vi "testCmdLineParser.vi"(8 "error in (no error)":errorcluster) -> (0 "error out":errorcluster)   [LabVIEW 2018]
uses:
  <vilib>/addons/_JKI Toolkits/Caraya/classes/Assert/Assert False.vi
  <vilib>/addons/_JKI Toolkits/Caraya/classes/Assert/Assert True.vi
  <vilib>/addons/_JKI Toolkits/Caraya/classes/Test/Test.lvclass
  <vilib>/addons/_JKI Toolkits/Caraya/classes/Assert/Assert.lvclass
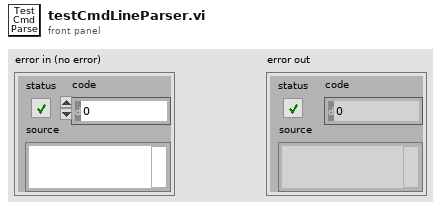
[diagram p1: front panel]
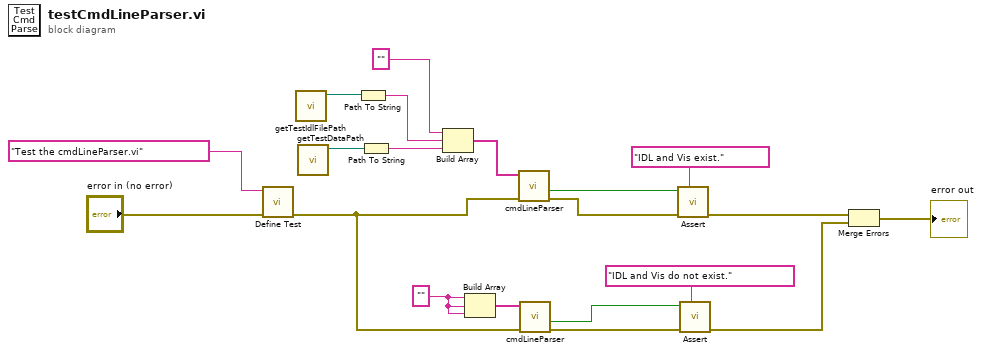
[diagram p0: block diagram]
diagram:
  w11 = ""
  n1 = call <vilib>:"Define Test.vi"("error in (no error)"="error in (no error)", "Label (VI Title)"="Test the cmdLineParser.vi") -> ("error out"=w9:errorcluster)  [unwired: 9 in]
  n2 = call "getTestIdlFilePath.vi"() -> ("testIdlPath"=w2:path)  [unwired: 11 in]
  n3 = call "getTestDataPath.vi"() -> ("testDataPath"=w1:path)  [unwired: 11 in]
  n4 = Path To String(path=w2) -> (string=w19:string)
  n5 = Path To String(path=w1) -> (string=w18:string)
  n6 = Build Array("", w19, w18) -> (w17:string[])
  n7 = Build Array(w11, w11, w11) -> (w10:string[])
  n8 = call "cmdLineParser.vi"("error in (no error)"=w9, "cmdLineArgs"=w17) -> ("error out"=w13:errorcluster, "filesExist"=w14:bool)  [unwired: 6 in, 2 out]
  n9 = call "cmdLineParser.vi"("error in (no error)"=w9, "cmdLineArgs"=w10) -> ("error out"=w8:errorcluster, "filesExist"=w3:bool)  [unwired: 6 in, 2 out]
  n10 = call-poly <vilib>:"Assert.vi"("Label"="IDL and Vis exist.", "error in (no error)"=w13, "True?"=w14) -> ("error out"=w6:errorcluster)  [unwired: 8 in]
  n11 = call-poly <vilib>:"Assert.vi"("Label"="IDL and Vis do not exist.", "error in (no error)"=w8, "False?"=w3) -> ("error out"=w5:errorcluster)  [unwired: 8 in]
  n12 = Merge Errors(w6, w5) -> (→"error out":errorcluster)
